vi "GetPosition.vi"(8 "error in (no error)":errorcluster, 11 "reference in":refnum<class "SceneObject.lvclass">) -> (0 "error out":errorcluster, 2 "Position":T1, 3 "reference out":refnum<class "SceneObject.lvclass">)   [LabVIEW 2010, in "RenderBase.lvlib" / "SceneObject.lvclass"]
uses:
  SceneObject.lvclass
  <vilib>/Utility/miscctls.llb/LV3DPointTypeDef.ctl
  SceneObject.lvclass/SceneObject.ctl
  <vilib>/picture/3D Picture Control/NI_3D Picture Control.lvlib
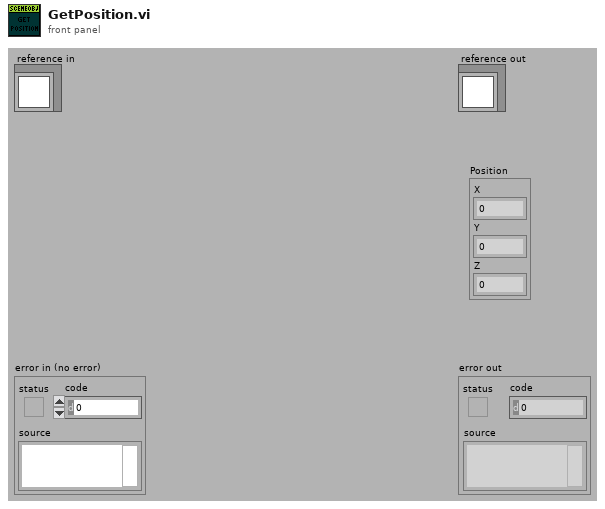
[diagram p1: front panel]
types:
  T1 = typedef "LV3DPointTypeDef.ctl" = cluster{"X":sgl, "Y":sgl, "Z":sgl}
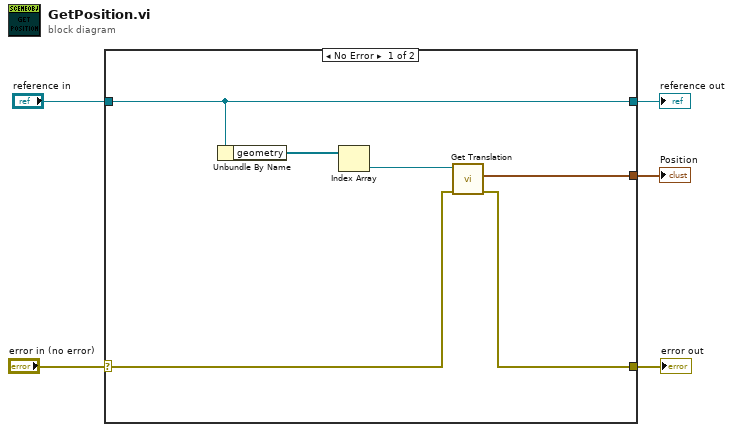
[diagram p0: block diagram]
diagram:
  n1 = case shown="No Error" "error in (no error)" {
    selector: "error in (no error)" -> [w8 w13]
    tunnel: [w7 w13] -> w4
    tunnel: [w11 w12] -> w2
    tunnel: "reference in" -> [w11 w12]
    tunnel: [w6 _] -> w1
    frame No Error {
      n2 = Unbundle By Name(w11) -> ("geometry"=w10:refnum<vi>[])
      n3 = Index Array(array=w10) -> (element=w9:refnum<vi>)  [unwired: 1 in]
      n4 = call <vilib>:"Get Translation.vi"("error in (no error)"=w8, "Scene Object"=w9) -> ("error out"=w7:errorcluster, "Transformation:Get Translation"=w6:cluster{"X":sgl, "Y":sgl, "Z":sgl})  [unwired: 7 in, 1 out]
    }
    frame Error {
    }
  }
  "error out" <- w4
  "reference out" <- w2
  "Position" <- w1
